vi "Excel Report - XY Graph Generation.vi"() -> ()   [LabVIEW 2023]
doc: "This example shows how to insert a XY graph into an Excel workbook and change the graph color attributes."
uses:
  <vilib>/Utility/NIReport.llb/Report Type.ctl
  <vilib>/Utility/NIReport.llb/NI_report.lvclass
  <vilib>/Utility/NIReport.llb/Excel/NI_Excel.lvclass
  <vilib>/Utility/NIReport.llb/NI_ReportGenerationCore.lvlib
panel:
  out "XY Graph":cluster{dbl[], dbl[]}(graph)
  # "Overview: This example shows how to insert a XY graph into an Excel worksheet and how to change the graph color attributes.\nRequirements: Report Generation Toolkit, Microsoft Excel\nInstructions:\nRun the VI."
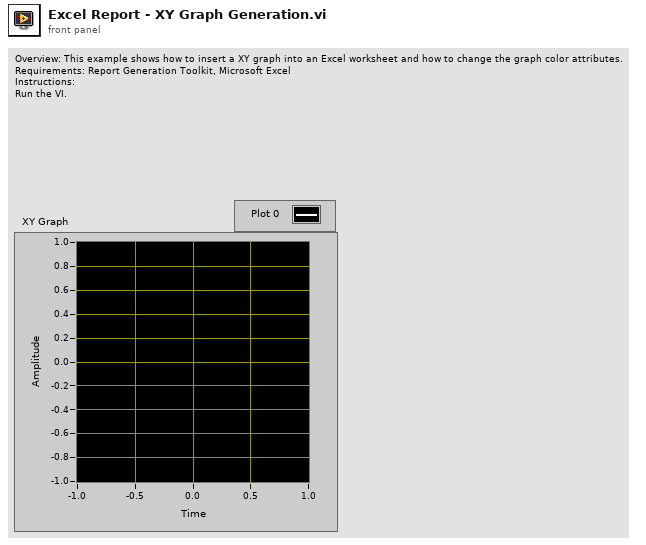
[diagram p1: front panel]
types:
  T1 = typedef "NI_ReportGenerationCore.lvlib/Report Type.ctl" = enum16{"HTML", "Word", "Excel"}
  T2 = cluster{"left":i32, "top":i32, "height":dbl, "width":dbl}
  T3 = cluster{"has major gridlines?":bool, "has minor gridlines?":bool, "major gridlines color":u32, "minor gridlines color":u32}
  T4 = cluster{"font style":string, "bold":bool, "italic":bool, "underline":bool, "size":sgl, "color":u32}
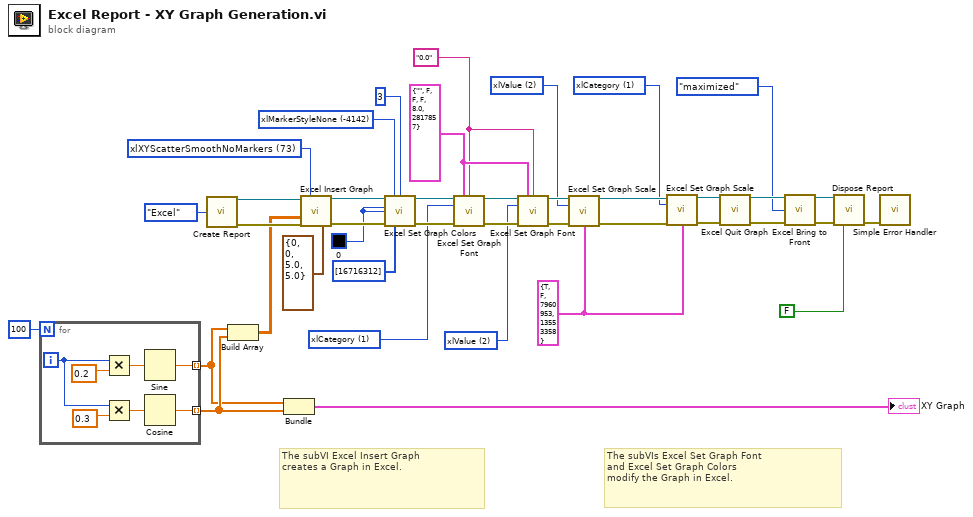
[diagram p0: block diagram]
diagram:
  w10 = "0.0" ("number format (general)")
  w16 = 1 items=["xlCategory"=1, "xlSeriesAxis"=3, "xlValue"=2] ("axis type")
  w19 = 2 items=["xlCategory"=1, "xlSeriesAxis"=3, "xlValue"=2] ("axis type")
  w15 = T3 {"has major gridlines?"=TRUE, "has minor gridlines?"=FALSE, "major gridlines color"=7960953, "minor gridlines color"=13553358} ("gridlines")
  w22 = 2 items=["xlCategory"=1, "xlSeriesAxis"=3, "xlValue"=2] ("axis type")
  w26 = 1 items=["xlCategory"=1, "xlSeriesAxis"=3, "xlValue"=2] ("axis type")
  w23 = T4 {"font style"="", "bold"=FALSE, "italic"=FALSE, "underline"=FALSE, "size"=8.0, "color"=2817857} ("axis font")
  w29 = u32 0 ("plot area color")
  w30 = -4142 items=["xlMarkerStyleAutomatic"=-4105, "xlMarkerStyleCircle"=8, "xlMarkerStyleDash"=-4115, "xlMarkerStyleDiamond"=2, "xlMarkerStyleDot"=-4118, "xlMarkerStyleNone"=-4142, "xlMarkerStylePicture"=-4147, "xlMarkerStylePlus"=9, "xlMarkerStyleSquare"=1, "xlMarkerStyleStar"=5, "xlMarkerStyleTriangle"=3, "xlMarkerStyleX"=-4168] ("marker style")
  w11 = 73 items=["xlColumnClustered"=51, "xlColumnStacked"=52, "xlColumnStacked100"=53, "xl3DColumnClustered"=54, "xl3DColumnStacked"=55, "xl3DColumnStacked100"=56, "xlBarClustered"=57, "xlBarStacked"=58, "xlBarStacked100"=59, "xl3DBarClustered"=60, "xl3DBarStacked"=61, "xl3DBarStacked100"=62, "xlLineStacked"=63, "xlLineStacked100"=64, "xlLineMarkers"=65, "xlLineMarkersStacked"=66, "xlLineMarkersStacked100"=67, "xlPieOfPie"=68, "xlPieExploded"=69, "xl3DPieExploded"=70, "xlBarOfPie"=71, "xlXYScatterSmooth"=72, "xlXYScatterSmoothNoMarkers"=73, "xlXYScatterLines"=74, "xlXYScatterLinesNoMarkers"=75, "xlAreaStacked"=76, "xlAreaStacked100"=77, "xl3DAreaStacked"=78, "xl3DAreaStacked100"=79, "xlDoughnutExploded"=80, "xlRadarMarkers"=81, "xlRadarFilled"=82, "xlSurface"=83, "xlSurfaceWireframe"=84, "xlSurfaceTopView"=85, "xlSurfaceTopViewWireframe"=86, "xlBubble"=15, "xlBubble3DEffect"=87, "xlStockHLC"=88, "xlStockOHLC"=89, "xlStockVHLC"=90, "xlStockVOHLC"=91, "xlCylinderColClustered"=92, "xlCylinderColStacked"=93, "xlCylinderColStacked100"=94, "xlCylinderBarClustered"=95, "xlCylinderBarStacked"=96, "xlCylinderBarStacked100"=97, "xlCylinderCol"=98, "xlConeColClustered"=99, "xlConeColStacked"=100, "xlConeColStacked100"=101, "xlConeBarClustered"=102, "xlConeBarStacked"=103, "xlConeBarStacked100"=104, "xlConeCol"=105, "xlPyramidColClustered"=106, "xlPyramidColStacked"=107, "xlPyramidColStacked100"=108, "xlPyramidBarClustered"=109, "xlPyramidBarStacked"=110, "xlPyramidBarStacked100"=111, "xlPyramidCol"=112, "xl3DColumn"=-4100, "xlLine"=4, "xl3DLine"=-4101, "xl3DPie"=-4102, "xlPie"=5, "xlXYScatter"=-4169, "xl3DArea"=-4098, "xlArea"=1, "xlDoughnut"=-4120, "xlRadar"=-4151] ("chart type")
  # "The subVIs Excel Set Graph Font \nand Excel Set Graph Colors \nmodify the Graph in Excel."
  # "The subVI Excel Insert Graph \ncreates a Graph in Excel."
  n1 = for {
    N: 100 -> [_]
    tunnel: [w46] -> w2 mode=indexing
    tunnel: [w45] -> w37 mode=indexing
    i -> [w41]
    n2 = Multiply(x=w41, y=0.2) -> (x*y=w43:dbl)
    n3 = Multiply(x=w41, y=0.3) -> (x*y=w42:dbl)
    n4 = Sine(x=w43) -> (sin(x)=w46:dbl)
    n5 = Cosine(x=w42) -> (cos(x)=w45:dbl)
  }
  n6 = call <vilib>:"Create Report.vi"("report type"=Report_Type."Excel" ("Report Type")) -> ("report out"=w39:refnum<class "NI_report.lvclass">, "error out"=w40:errorcluster)  [unwired: 13 in]
  n7 = Build Array(w2, w37) -> (w36:dbl[][])
  n8 = Bundle(w2, w37) -> (→"XY Graph":cluster{dbl[], dbl[]})  [unwired: 1 in]
  n9 = call <vilib>:"Excel Insert Graph.vi"("report in"=w39, "graph type (col clustered)"=w11, "data"=w36, "error in (no error)"=w40, "position/size"=T2 {"left"=0, "top"=0, "height"=5.0, "width"=5.0}) -> ("report out"=w33:refnum<class "NI_report.lvclass">, "error out"=w34:errorcluster)  [unwired: 9 in]
  n10 = call <vilib>:"Excel Set Graph Colors.vi"("report in"=w33, "marker style (none)"=w30, "weight (1)"=i16 3 ("weight"), "graph area color (w)"=w29, "plot area color (w)"=w29, "error in (no error)"=w34, "plot colors"=u32[] [16716312]) -> ("report out"=w27:refnum<class "NI_report.lvclass">, "error out"=w28:errorcluster)  [unwired: 7 in]
  n11 = call <vilib>:"Excel Set Graph Font.vi"("report in"=w27, "axis font"=w23, "number format (general)"=w10, "axis type (xlCategory)"=w26, "error in (no error)"=w28) -> ("report out"=w24:refnum<class "NI_report.lvclass">, "error out"=w25:errorcluster)  [unwired: 9 in]
  n12 = call <vilib>:"Excel Set Graph Font.vi"("report in"=w24, "axis font"=w23, "number format (general)"=w10, "axis type (xlCategory)"=w22, "error in (no error)"=w25) -> ("report out"=w20:refnum<class "NI_report.lvclass">, "error out"=w21:errorcluster)  [unwired: 9 in]
  n13 = call <vilib>:"Excel Set Graph Scale.vi"("report in"=w20, "axis type (xlCategory)"=w19, "error in (no error)"=w21, "gridlines"=w15) -> ("report out"=w17:refnum<class "NI_report.lvclass">, "error out"=w18:errorcluster)  [unwired: 10 in]
  n14 = call <vilib>:"Excel Set Graph Scale.vi"("report in"=w17, "axis type (xlCategory)"=w16, "error in (no error)"=w18, "gridlines"=w15) -> ("report out"=w14:refnum<class "NI_report.lvclass">, "error out"=w13:errorcluster)  [unwired: 10 in]
  n15 = call <vilib>:"Excel Quit Graph.vi"("report in"=w14, "error in (no error)"=w13) -> ("report out"=w8:refnum<class "NI_report.lvclass">, "error out"=w9:errorcluster)  [unwired: 12 in]
  n16 = call <vilib>:"Excel Bring to Front.vi"("report in"=w8, "window state (maximized)"=enum16{"maximized", "minimized", "normal"}."maximized", "error in (no error)"=w9) -> ("report out"=w5:refnum<class "NI_report.lvclass">, "error out"=w6:errorcluster)  [unwired: 11 in]
  n17 = call-dynamic "Dispose Report.vi"("report in"=w5, "error in (no error)"=w6, "close report? (T)"=FALSE ("Close Report? (T)")) -> ("error out"=w4:errorcluster)  [unwired: 12 in]
  n18 = call <vilib>:"Simple Error Handler.vi"("error in (no error)"=w4) -> ()  [unwired: 4 in, 5 out]
